vi "Main.vi"() -> ()   [LabVIEW 2018]
uses:
  Initialize/CreateQueue/AllDataQueue.ctl
  Initialize/CreateQueue/SocketQueue.ctl
  Initialize/CreateQueue/LogDataQueue.ctl
  Initialize/CreateQueue/ProDataQueue.ctl
  ProData/SettingData.ctl
  socket/socket.ctl
  Initialize/Setting/DA.ctl
  Initialize/Setting/AD.ctl
  ProData/prodatascan.ctl
  Support/Data.ctl
  <vilib>/DAQmx/read.llb/DAQmx Read (Analog Wfm 1Chan NSamp).vi
  <vilib>/DAQmx/write.llb/DAQmx Write (Analog DBL 1Chan 1Samp).vi
  <vilib>/DAQmx/create/channels.llb/DAQmx Create Channel (AI-Voltage-Basic).vi
  <vilib>/DAQmx/configure/timing.llb/DAQmx Timing (Sample Clock).vi
  <vilib>/DAQmx/miscellaneous.llb/DAQmx Fill In Error Info.vi
  <vilib>/DAQmx/create/channels.llb/DAQmx Create Channel (AO-Voltage-Basic).vi
panel:
  out "设备名":string
  in  "选项卡控件":enum32{"Setting", "Chart"}(tab)
  in  "timeout":i16=-1
  in  "标准差倍数":dbl=7.0
  in  "normal":string="1"
  in  "每通道采样率":u16=60
  in  "电压最大值":u16=5
  in  "电压最小值":i16=-5
  in  "采样率":u16=60000
  in  "接线方式":i32(ring)=10106 items=["默认"=-1, "RSE"=10083, "NRSE"=10078, "差分"=10106, "伪差分"=12529]
  in  "采样模式":i32(ring)=10123 items=["有限采样"=10178, "连续采样"=10123, "硬件定时单点"=12522]
  in  "DA电压最大值":dbl=10.0
  in  "DA电压最小值":dbl=-10.0
  in  "地址":string="8.131.237.84"
  out "选择通道AD  2":tag="USB_6211_2/ai1"
  out "连接状态":string="连接成功"
  in  "adjust":dbl=0.1
  out "波形图表":i32(graph)
  out "nvpai":dbl
  out "max":dbl
  out "min":dbl
  in  "等待时间（毫秒）":u32=15
  out "ADchart":dbl(graph)
  out "DAchart":dbl(graph)
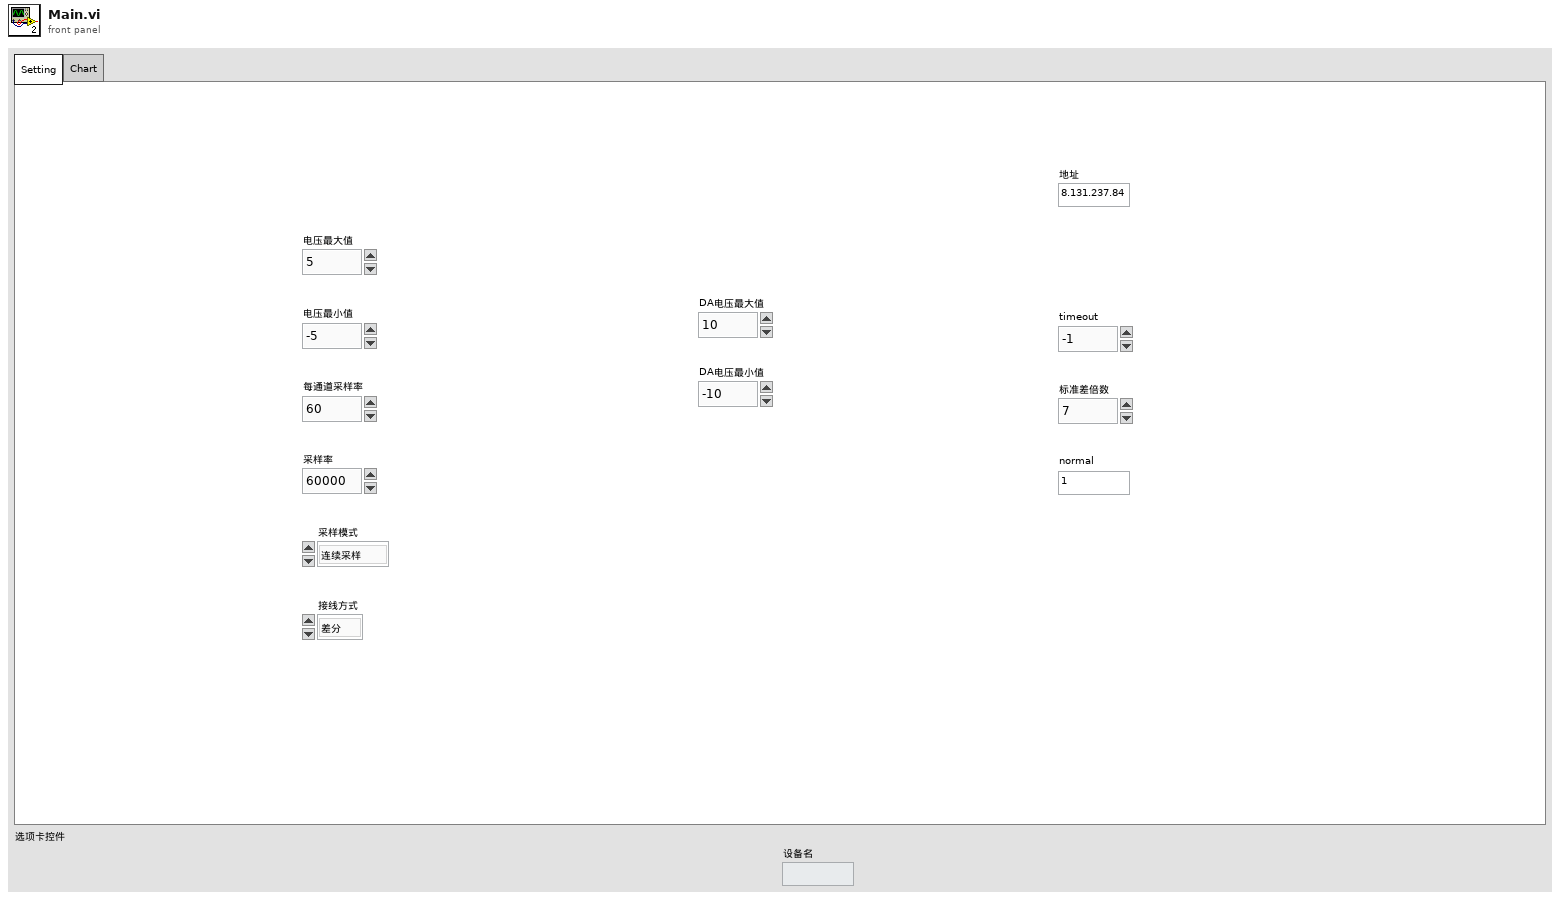
[diagram p1: front panel]
types:
  T1 = typedef "socket.ctl" = cluster{"端口":u16, "timeout":u16, "标准差倍数":dbl, "address":string, "abnormal":string}
  T2 = typedef "DA.ctl" = cluster{"电压最大值":dbl, " 电压最小值":dbl, "选择通道DA ":tag}
  T3 = typedef "AD.ctl" = cluster{"电压最大值":u16, " 电压最小值":i16, " 采样率":u16, "每通道采样率":u16, "采样模式":i32, "接线方式":i32, "source":tag, "选择通道AD ":tag}
  T4 = typedef "Data.ctl" = cluster{"SynQueue":cluster{"SocketQueue":T5, "LogQueue":T6, " DA":refnum<queue>, "ProQueue":T7}, "Error":cluster{"错误输出 2":errorcluster}, "SettingData":T8}
  T5 = typedef "SocketQueue.ctl" = cluster{"ADSTDqueue ":refnum<queue>, "SocketADExceptionqueue":refnum<queue>, "  SocketAD":refnum<queue>}
  T6 = typedef "LogDataQueue.ctl" = cluster{"RunningADqueue":refnum<queue>, "Compensatequeue":refnum<queue>, " RunningDAqueue":refnum<queue>, " RunMin":refnum<queue>}
  T7 = typedef "ProDataQueue.ctl" = cluster{"buffer ":refnum<queue>, " StimeADqueue":refnum<queue>, "  MtimeADqueue":refnum<queue>}
  T8 = typedef "SettingData.ctl" = cluster{"socket":T1, "DA":T2, "AD":T3, "prodatascan":T9}
  T9 = typedef "prodatascan.ctl" = cluster{"max":dbl, "min":dbl, " nvpai":dbl, "初始化数组":dbl[]}
  T10 = typedef "AllDataQueue.ctl" = cluster{"SocketQueue":T5, "LogQueue":T6, " DA":refnum<queue>, "ProQueue":T7}
  T11 = cluster{"max":dbl, "min":dbl, " nvpai":dbl, "初始化数组":dbl[]}
  T12 = cluster{"SocketQueue":T5, "LogQueue":T6, " DA":refnum<queue>, "ProQueue":T7}
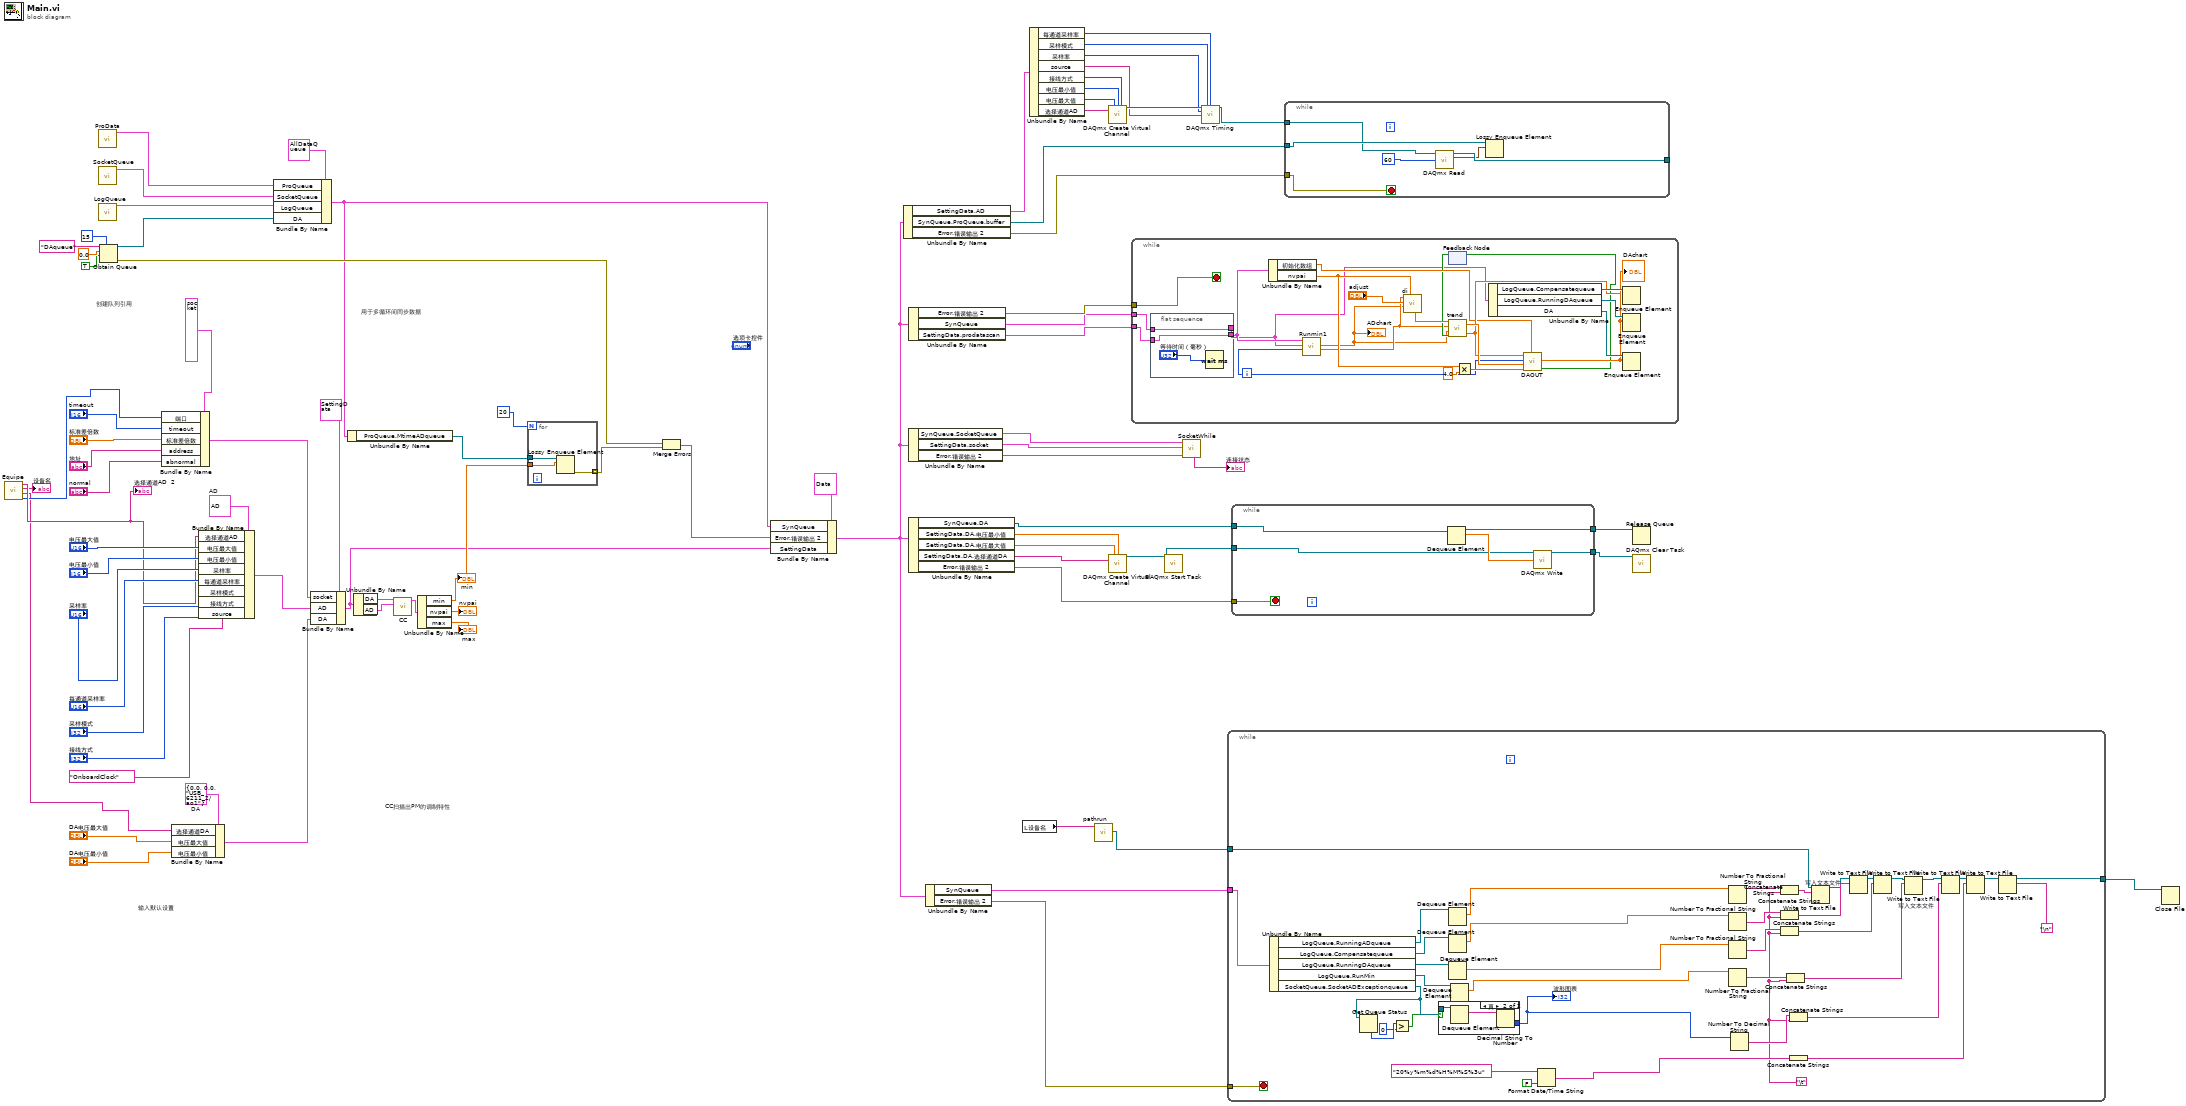
[diagram p0: block diagram]
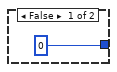
[diagram p2: hidden frame]
diagram:
  w8 = T2 {"电压最大值"=0.0, " 电压最小值"=0.0, "选择通道DA "="USB_6211_2/ao1"}  # DA
  w9 = T3 {"电压最大值"=10013, " 电压最小值"=10013, " 采样率"=10013, "每通道采样率"=10013, "采样模式"=10123, "接线方式"=10106, "source"="OnboardClock", "选择通道AD "="USB_6211_2/ai1"}  # AD
  # "CC扫描出PM的调制特性"
  # "输入默认设置"
  # "用于多循环间同步数据"
  # "创建队列引用"
  n1 = call "Equipe.vi"() -> ("port"=w3:i32, "DA"=w2:string, "设备名"=→"设备名":string, "AD"=w5:string)  [unwired: 8 in]
  "选择通道AD  2" <- w5
  n2 = call "ProData.vi"() -> ("ProDataQueue"=w74:T7)  [unwired: 11 in]
  n3 = call "SocketQueue.vi"() -> ("SocketQueue"=w76:T5)  [unwired: 11 in]
  n4 = call "LogQueue.vi"() -> ("LogQueue"=w75:T6)  [unwired: 11 in]
  n5 = Obtain Queue(max queue size (-1, unlimited)=15 ("队列最大值（-1，无限）"), name (unnamed)="DAqueue" ("名称（未命名）"), element data type=0.0, create if not found? (T)=TRUE ("如未找到则创建？(T)")) -> (queue out=w77:refnum<queue>, error out=w52:errorcluster)  [unwired: 1 in, 1 out]
  n6 = Bundle By Name(cluster=T1 {"端口"=10013, "timeout"=10013, "标准差倍数"=0.0, "address"="{\"ad\":1}", "abnormal"="{\"ad\":0}"} ("socket"), "端口"=w3, "timeout"="timeout", "标准差倍数"="标准差倍数", "address"="地址", "abnormal"="normal") -> (w63:T1)
  n7 = Bundle By Name(cluster=w8, "选择通道DA"=w2, "电压最大值"="DA电压最大值", "电压最小值"="DA电压最小值") -> (w59:T2)
  n8 = Bundle By Name(cluster=w9, "选择通道AD"=w5, "电压最大值"="电压最大值", "电压最小值"="电压最小值", "采样率"="采样率", "每通道采样率"="每通道采样率", "采样模式"="采样模式", "接线方式"="接线方式", "source"=tag "OnboardClock") -> (w58:T3)
  n9 = Bundle By Name(cluster=T10 {"SocketQueue"={"ADSTDqueue "=refnum, "SocketADExceptionqueue"=refnum, "  SocketAD"=refnum}, "LogQueue"={"RunningADqueue"=refnum, "Compensatequeue"=refnum, " RunningDAqueue"=refnum, " RunMin"=refnum}, " DA"=refnum, "ProQueue"={"buffer "=refnum, " StimeADqueue"=refnum, "  MtimeADqueue"=refnum}}, "ProQueue"=w74, "SocketQueue"=w76, "LogQueue"=w75, "DA"=w77) -> (w40:T10)
  n10 = Bundle By Name(cluster=T8 {"socket"={"端口"=10013, "timeout"=10013, "标准差倍数"=0.0, "address"="{\"ad\":1}", "abnormal"="{\"ad\":0}"}, "DA"={"电压最大值"=0.0, " 电压最小值"=0.0, "选择通道DA "="USB_6211_2/ao1"}, "AD"={"电压最大值"=10013, " 电压最小值"=10013, " 采样率"=10013, "每通道采样率"=10013, "采样模式"=10123, "接线方式"=10106, "source"="OnboardClock", "选择通道AD "="USB_6211_2/ai1"}, "prodatascan"={"max"=0.0, "min"=0.0, " nvpai"=0.0, "初始化数组"=[]}} ("SettingData"), "socket"=w63, "AD"=w58, "DA"=w59) -> (w46:T8)
  n11 = Unbundle By Name(w40) -> ("ProQueue.MtimeADqueue"=w54:refnum<queue>)
  n12 = Unbundle By Name(w46) -> ("DA"=w56:T2, "AD"=w57:T3)
  n13 = call "CC.vi"("AD"=w57, "DA"=w56) -> ("prodatascan"=w47:T11)  [unwired: 8 in, 1 out]
  n14 = Unbundle By Name(w47) -> ("min"=w55:dbl, "nvpai"=→"nvpai":dbl, "max"=→"max":dbl)
  "min" <- w55
  n15 = for {
    N: 20 -> [_]
    tunnel: w54 -> [w85]
    tunnel: w55 -> [w84]
    tunnel: [w83] -> w51 mode=indexing
    n16 = Lossy Enqueue Element(queue=w85, element=w84) -> (error out=w83:errorcluster)  [unwired: 1 in, 3 out]
  }
  n17 = Merge Errors(w52, w51) -> (w30:errorcluster)
  n18 = Bundle By Name(cluster=T4 {"SynQueue"={"SocketQueue"={"ADSTDqueue "=refnum, "SocketADExceptionqueue"=refnum, "  SocketAD"=refnum}, "LogQueue"={"RunningADqueue"=refnum, "Compensatequeue"=refnum, " RunningDAqueue"=refnum, " RunMin"=refnum}, " DA"=refnum, "ProQueue"={"buffer "=refnum, " StimeADqueue"=refnum, "  MtimeADqueue"=refnum}}, "Error"={"错误输出 2"={"status"=FALSE, "code"=0, "source"=""}}, "SettingData"={"socket"={"端口"=0, "timeout"=0, "标准差倍数"=0.0, "address"="{\"ad\":1}", "abnormal"="{\"ad\":0}"}, "DA"={"电压最大值"=0.0, " 电压最小值"=0.0, "选择通道DA "="USB_6211_2/ao1"}, "AD"={"电压最大值"=10013, " 电压最小值"=10013, " 采样率"=10013, "每通道采样率"=10013, "采样模式"=10123, "接线方式"=10106, "source"="OnboardClock", "选择通道AD "="USB_6211_2/ai1"}, "prodatascan"={"max"=0.0, "min"=0.0, " nvpai"=0.0, "初始化数组"=[]}}}, "SynQueue"=w40, "Error.错误输出 2"=w30, "SettingData"=w46) -> (w15:T4)
  n19 = Unbundle By Name(w15) -> ("SettingData.AD"=w18:T3, "SynQueue.ProQueue.buffer"=w28:refnum<queue>, "Error.错误输出 2"=w29:errorcluster)
  n20 = Unbundle By Name(w15) -> ("Error.错误输出 2"=w43:errorcluster, "SynQueue"=w41:T12, "SettingData.prodatascan"=w42:T9)
  n21 = Unbundle By Name(w15) -> ("SynQueue.SocketQueue"=w44:T5, "SettingData.socket"=w7:T1, "Error.错误输出 2"=w45:errorcluster)
  n22 = Unbundle By Name(w15) -> ("SynQueue.DA"=w34:refnum<queue>, "SettingData.DA.电压最小值"=w37:dbl, "SettingData.DA.电压最大值"=w33:dbl, "SettingData.DA.选择通道DA"=w38:tag, "Error.错误输出 2"=w39:errorcluster)
  n23 = Unbundle By Name(w15) -> ("SynQueue"=w14:T12, "Error.错误输出 2"=w13:errorcluster)
  n24 = local read "设备名"() -> (w1:string)
  n25 = Unbundle By Name(w18) -> ("每通道采样率"=w19:u16, "采样模式"=w20:i32, "采样率"=w21:u16, "source"=w22:tag, "接线方式"=w27:i32, "电压最小值"=w26:i16, "电压最大值"=w25:u16, "选择通道AD"=w24:tag)
  n26 = call "pathrun.vi"("时间格式字符串(%c)"=w1) -> ("引用句柄输出"=w16:refnum<file>)  [unwired: 10 in]
  n27 = call-poly <vilib>:"DAQmx Create Virtual Channel.vi"("maximum value"=w25, "minimum value"=w26, "input terminal configuration"=w27, "physical channels"=w24) -> ("task out"=w23:refnum<k21>)  [unwired: 10 in, 1 out]
  n28 = call-poly <vilib>:"DAQmx Create Virtual Channel.vi"("maximum value"=w33, "minimum value"=w37, "physical channels"=w38) -> ("task out"=w36:refnum<k21>)  [unwired: 11 in, 1 out]
  n29 = while {
    tunnel: w43 -> [w105]
    tunnel: w41 -> [w87]
    tunnel: w42 -> [w89]
    i -> [w93]
    stop <- w105 stop-if-true
    n30 = flat-sequence {
      tunnel: w89 -> [w109]
      tunnel: [w109] -> w88
      tunnel: w87 -> [w108]
      tunnel: [w108] -> w86
      frame #0 {
        n31 = Wait (ms)(milliseconds to wait="等待时间（毫秒）") -> ()  [unwired: 1 out]
      }
    }
    n32 = Unbundle By Name(w88) -> ("初始化数组"=w96:dbl[], "nvpai"=w92:dbl)
    n33 = call "Runmin1.vi"("循环次数 i"=w93, "Queue1"=w86, "prodatascan"=w88) -> ("runMin"=w91:dbl, "AD"=w90:dbl)  [unwired: 7 in]
    "ADchart" <- w90
    n34 = call "di.vi"("RunMin"=w91, "adjust"="adjust", "AD"=w90, "Nvpai"=w92) -> ("Compensate1"=w106:dbl)  [unwired: 6 in]
    n35 = feedback #1() -> (w94:bool)  [unwired: 1 in]
    n36 = call "trend.vi"("jumpBool"=w94, "AD"=w90, "runMin"=w91, "Compensate1"=w106) -> ("Compensate1Out"=w97:dbl, "changeSymbol"=w98:dbl)
    n37 = Multiply(x=w92, y=4.0) -> (x*y=w99:dbl)
    n38 = Unbundle By Name(w86) -> ("LogQueue.Compensatequeue"=w104:refnum<queue>, "LogQueue.RunningDAqueue"=w103:refnum<queue>, "DA"=w101:refnum<queue>)
    n39 = call "DAOUT.vi"("maxInitial数组"=w96, "maxInitialVoltage"=w99, "changeSymbol"=w98, "running recycle counter"=w93, "compensate"=w97) -> ("jump symbol"=w95:bool, "real running DA output"=w100:dbl)  [unwired: 5 in]
    "DAchart" <- w100
    n40 = feedback-in #1(w95) -> ()
    n41 = Enqueue Element(queue=w104, element=w97) -> ()  [unwired: 2 in, 3 out]
    n42 = Enqueue Element(queue=w103, element=w100) -> ()  [unwired: 2 in, 3 out]
    n43 = Enqueue Element(queue=w101, element=w100) -> ()  [unwired: 2 in, 3 out]
  }
  n44 = call <vilib>:"DAQmx Start Task.vi"("task/channels in"=w36) -> ("task out"=w35:refnum<k21>)  [unwired: 13 in, 1 out]
  n45 = call "SocketWhile.vi"("error out"=w45, "socket 2"=w7, "SocketQueue"=w44) -> ("socket"=→"连接状态":string)  [unwired: 8 in]
  n46 = call-poly <vilib>:"DAQmx Timing.vi"("task/channels in"=w23, "sample mode"=w20, "samples per channel"=w19, "rate"=w21, "source"=w22) -> ("task out"=w17:refnum<k21>)  [unwired: 9 in, 1 out]
  n47 = while {
    tunnel: w13 -> [w144]
    tunnel: [w114] -> w12
    tunnel: w16 -> [w113]
    tunnel: w14 -> [w111]
    stop <- w144 stop-if-true
    w112 = "\t"
    n48 = Unbundle By Name(w111) -> ("LogQueue.RunningADqueue"=w143:refnum<queue>, "LogQueue.Compensatequeue"=w147:refnum<queue>, "LogQueue.RunningDAqueue"=w146:refnum<queue>, "LogQueue.RunMin"=w145:refnum<queue>, "SocketQueue.SocketADExceptionqueue"=w142:refnum<queue>)
    n49 = Get Queue Status(queue=w142) -> (# elements in queue=w141:i32)  [unwired: 2 in, 7 out]
    n50 = Greater?(x=w141, y=0) -> (0:w139:bool)
    n51 = case shown="真" w139 {
      tunnel: [0 w152] -> w119
      tunnel: w142 -> [_ w151]
      frame False {
      }
      frame True {
        n52 = Dequeue Element(queue=w151) -> (element=w153:string)  [unwired: 2 in, 3 out]
        n53 = Decimal String To Number(string=w153) -> (number=w152:i32)  [unwired: 2 in, 1 out]
      }
    }
    "波形图表" <- w119
    n54 = Dequeue Element(queue=w143) -> (element=w129:dbl)  [unwired: 2 in, 3 out]
    n55 = Dequeue Element(queue=w147) -> (element=w128:dbl)  [unwired: 2 in, 3 out]
    n56 = Dequeue Element(queue=w146) -> (element=w127:dbl)  [unwired: 2 in, 3 out]
    n57 = Dequeue Element(queue=w145) -> (element=w121:dbl)  [unwired: 2 in, 3 out]
    n58 = Format Date/Time String(time format string (%c)="20%y%m%d%H%M%S%3u" ("时间格式字符串(%c)"), UTC format=FALSE ("UTC格式")) -> (date/time string=w117:string)  [unwired: 1 in]
    n59 = Number To Fractional String(number=w129) -> (F-format string=w134:string)  [unwired: 3 in]
    n60 = Number To Fractional String(number=w128) -> (F-format string=w136:string)  [unwired: 3 in]
    n61 = Number To Fractional String(number=w127) -> (F-format string=w137:string)  [unwired: 3 in]
    n62 = Number To Fractional String(number=w121) -> (F-format string=w122:string)  [unwired: 3 in]
    n63 = Number To Decimal String(number=w119) -> (decimal integer string=w118:string)  [unwired: 1 in]
    n64 = Concatenate Strings(w134, w112) -> (w131:string)
    n65 = Concatenate Strings(w136, w112) -> (w133:string)
    n66 = Concatenate Strings(w137, w112) -> (w138:string)
    n67 = Concatenate Strings(w122, w112) -> (w120:string)
    n68 = Concatenate Strings(w118, w112) -> (w116:string)
    n69 = Concatenate Strings(w117) -> (w115:string)
    n70 = Write to Text File "写入文本文件"(file (use dialog)=w113, text=w131) -> (refnum out=w132:refnum<file>)  [unwired: 2 in, 2 out]
    n71 = Write to Text File(file (use dialog)=w132, text=w133) -> (refnum out=w135:refnum<file>)  [unwired: 2 in, 2 out]
    n72 = Write to Text File(file (use dialog)=w135, text=w138) -> (refnum out=w124:refnum<file>)  [unwired: 2 in, 2 out]
    n73 = Write to Text File "写入文本文件"(file (use dialog)=w124, text=w120) -> (refnum out=w125:refnum<file>)  [unwired: 2 in, 2 out]
    n74 = Write to Text File(file (use dialog)=w125, text=w116) -> (refnum out=w126:refnum<file>)  [unwired: 2 in, 2 out]
    n75 = Write to Text File(file (use dialog)=w126, text=w115) -> (refnum out=w123:refnum<file>)  [unwired: 2 in, 2 out]
    n76 = Write to Text File(file (use dialog)=w123, text="\n") -> (refnum out=w114:refnum<file>)  [unwired: 2 in, 2 out]
  }
  n77 = while {
    tunnel: [w159] -> w31
    tunnel: [w158] -> w32
    tunnel: w34 -> [w155]
    tunnel: w39 -> [w156]
    tunnel: w35 -> [w154]
    stop <- w156 stop-if-true
    n78 = Dequeue Element(queue=w155) -> (queue out=w158:refnum<queue>, element=w157:dbl)  [unwired: 2 in, 2 out]
    n79 = call-poly <vilib>:"DAQmx Write.vi"("task/channels in"=w154, "data"=w157) -> ("task out"=w159:refnum<k21>)  [unwired: 11 in, 2 out]
  }
  n80 = while {
    tunnel: [w165] -> _
    tunnel: w28 -> [w162]
    tunnel: w29 -> [w161]
    tunnel: w17 -> [w160]
    stop <- w161 stop-if-true
    n81 = call-poly <vilib>:"DAQmx Read.vi"("task/channels in"=w160, "number of samples per channel"=60) -> ("task out"=w165:refnum<k21>, "data"=w164:waveform(dbl))  [unwired: 11 in, 1 out]
    n82 = Lossy Enqueue Element(queue=w162, element=w164) -> ()  [unwired: 1 in, 4 out]
  }
  n83 = Release Queue(queue=w32) -> ()  [unwired: 2 in, 3 out]
  n84 = call <vilib>:"DAQmx Clear Task.vi"("task in"=w31) -> ()  [unwired: 14 in, 1 out]
  n85 = Close File(refnum=w12) -> ()  [unwired: 1 in, 2 out]
